vi "SetControlsIndicators.vi"(6 "VI Index":i32, 9 "Indicators":string[][](array[string]), 10 "Controls":string[][](array[string]), 11 "Data In":T1[](array[typedef])) -> (3 "Data Out":T1[](array[typedef]))   [LabVIEW 2016, in "update vi properties.lvlib"]
uses:
  update vi properties.lvlib
  Cluster_Data.ctl
  <vilib>/picture/picture.llb/imagedata.ctl
panel:
  # "Connector Pane"
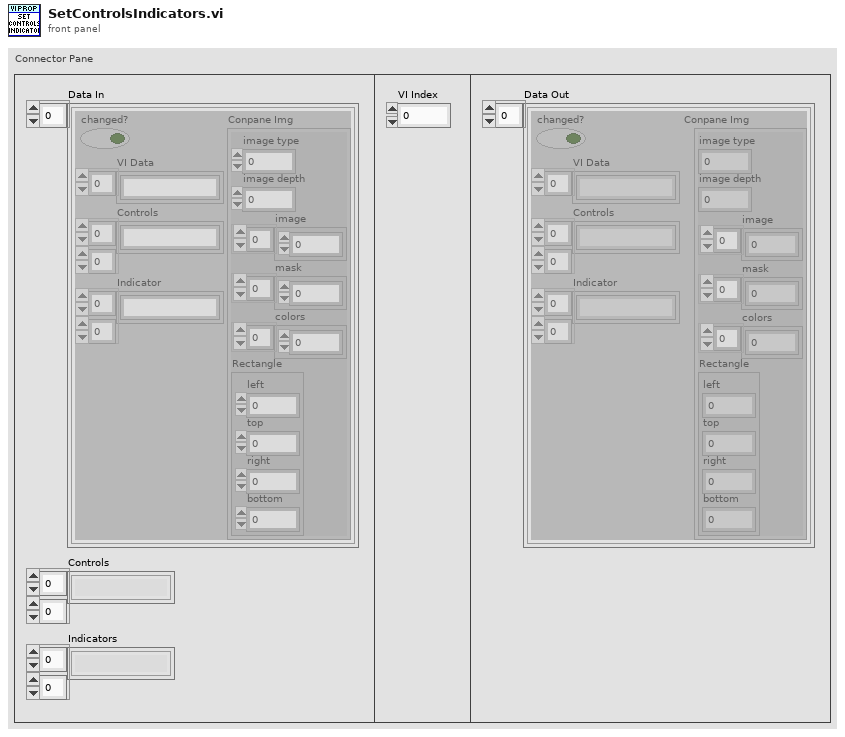
[diagram p1: front panel]
types:
  T1 = typedef "update vi properties.lvlib/Cluster_Data.ctl" = cluster{"changed?":bool, "VI Data":string[], "Controls":string[][], "Indicator":string[][], "Conpane Img":T2}
  T2 = typedef "imagedata.ctl" = cluster{"image type":i32, "image depth":i32, "image":u8[], "mask":u8[], "colors":u32[], "Rectangle":cluster{"left":i16, "top":i16, "right":i16, "bottom":i16}}
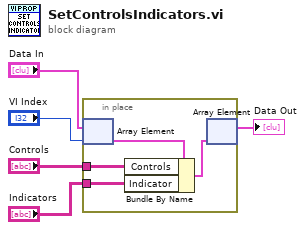
[diagram p0: block diagram]
diagram:
  n1 = in-place {
    in-place-border: "Controls" -> [w8]
    in-place-border: "Indicators" -> [w7]
    n2 = in-place-array #1("Data In", "VI Index") -> (w9:T1)
    n3 = Bundle By Name(cluster=w9, "Controls"=w8, "Indicator"=w7) -> (w6:T1)
    n4 = in-place-array #1(w6) -> (→"Data Out":T1[])  [unwired: 1 out]
  }
